vi "PythonNode_getlog.vi"() -> ()   [LabVIEW 2022 SP3]
doc: "This example demonstrates how to call a Python function and pass doubles as arguments. It uses a python function to compute the sum of two doubles."
panel:
  out "return value":dbl
  in  "module path":path
  out "error out":errorcluster
  in  "error in (no error)":errorcluster
  # "Overview: Demonstrates how to call a Python function and pass doubles as arguments.\nRequirements: Python 3.6, 3.7, 3.8 or 3.9 with the same bitness as LabVIEW.\nInstructions:\n1. Set the Python version to the version of Python you want to execute code in.\n2. Run the VI. You should see the result of adding \"a\" and \"b\" in the indicator \"a + b\".\n3. See comments on the block diagram of this VI and in \"ExamplePythonModule.py\" for more information about how the call python node passes arguments and handles return values."
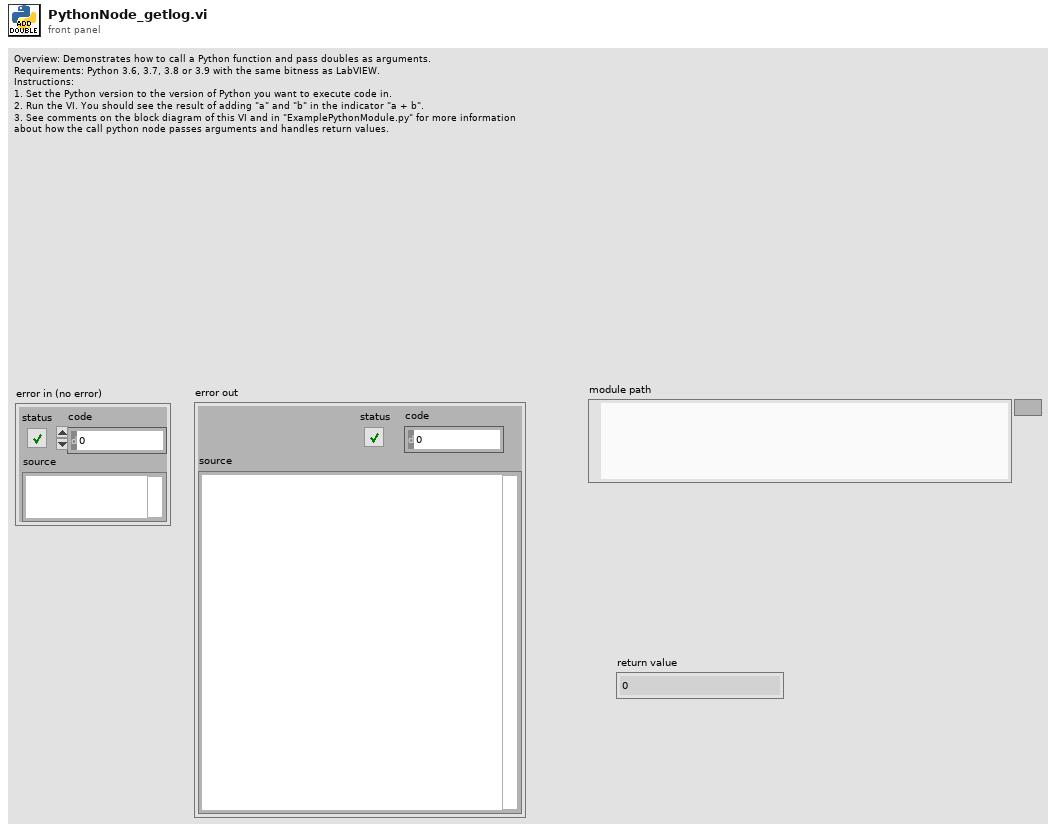
[diagram p1: front panel]
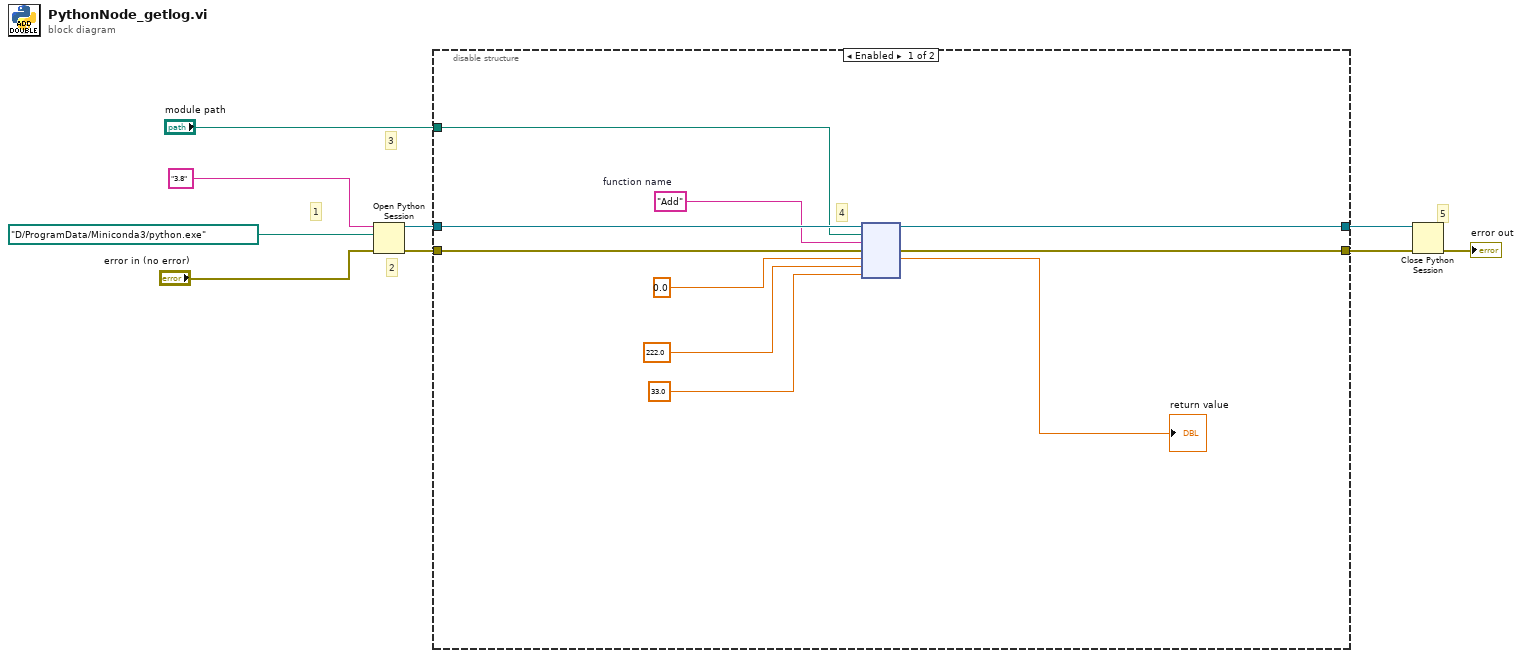
[diagram p0: block diagram]
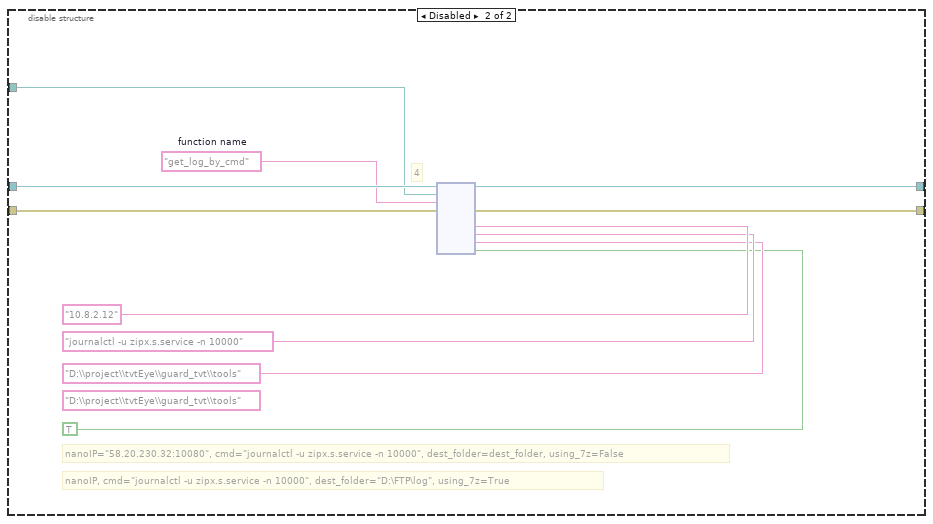
[diagram p2: hidden frame]
diagram:
  # "5"
  # "2"
  # "3"
  # "1"
  n1 = Open Python Session(python version="3.8" ("Python version"), python path=path "D:/ProgramData/Miniconda3/python.exe" ("Python path"), 3:"error in (no error)") -> (session out=w8:refnum<k35>, error out=w7:errorcluster)
  n2 = disable-structure shown="Enabled" {
    disable-tunnel: w8 -> [w19 w29]
    disable-tunnel: w7 -> [w18 w28]
    disable-tunnel: [w16 w26] -> w6
    disable-tunnel: [w15 w25] -> w5
    disable-tunnel: "module path" -> [w14 w24]
    frame Enabled {
      w17 = "Add"  # function name
      # "4"
      n3 = node(w19, w14, w17, w18, 0.0 ("a"), 222.0 ("a"), 33.0 ("a")) -> (w16:refnum<k35>, w15:errorcluster, →"return value":dbl)  [unwired: 2 in, 2 out]
    }
    frame Disabled {
      (unwired) "D:\\project\\tvtEye\\guard_tvt\\tools"
      w27 = "get_log_by_cmd"  # function name
      # "nanoIP=\"58.20.230.32:10080\", cmd=\"journalctl -u zipx.s.service -n 10000\", dest_folder=dest_folder, using_7z=False"
      # "nanoIP, cmd=\"journalctl -u zipx.s.service -n 10000\", dest_folder=\"D:\\FTP\\log\", using_7z=True"
      # "4"
      n4 = node(w29, w24, w27, w28, "10.8.2.12", "journalctl -u zipx.s.service -n 10000", "D:\\project\\tvtEye\\guard_tvt\\tools", TRUE) -> (w26:refnum<k35>, w25:errorcluster)  [unwired: 6 in, 2 out]
    }
  }
  n5 = Close Python Session(session in=w6, error in=w5) -> (11:→"error out":errorcluster)
